vi "Configure IQ Attenuation.vi"(6 "Optimization Bandwidth (1 Msps)":dbl=1000000.0, 8 "error in (no error)":errorcluster, 9 "Manual Level (0.4 V)":dbl=0.4, 10 "I/Q Input Level Method (0: Default)":u16(ring) items=["Default", "Manual", "Measurement"], 11 "VISA resource name":refnum<visa-resource-name>) -> (0 "error out":errorcluster, 3 "VISA resource name out":refnum<visa-resource-name>)   [LabVIEW 2014, in "Agilent PSG MXG Series.lvlib"]
doc: "Configures attenuation mode, attenuation level, external I/Q input level and bandwidth.\n\n<B>Notes:</B>\n(1) This VI is valid only in E8267C, E8267D."
uses:
  Agilent PSG MXG Series.lvlib
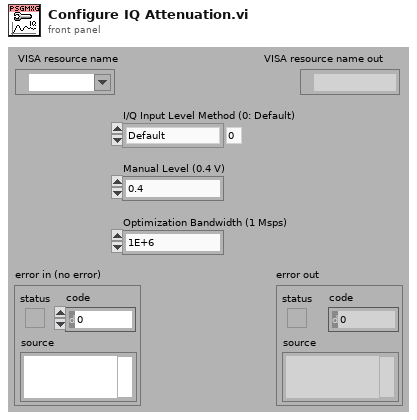
[diagram p1: front panel]
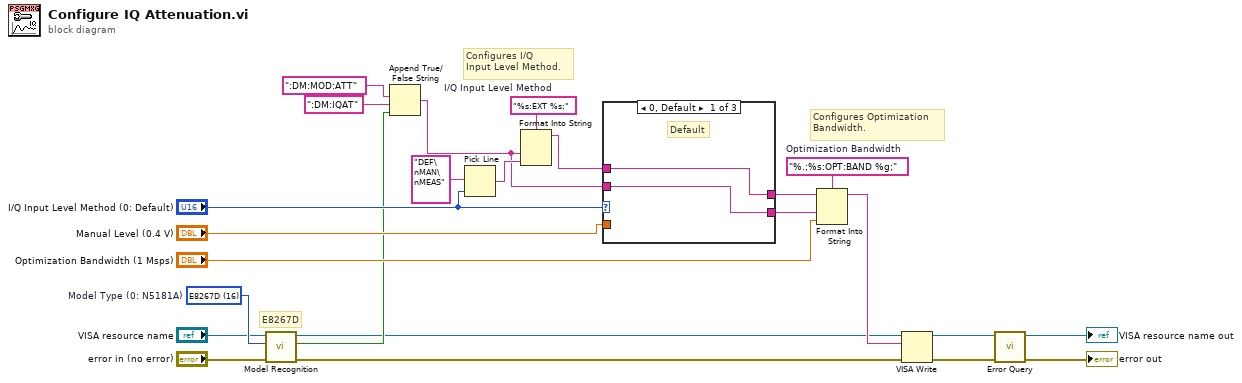
[diagram p0: block diagram]
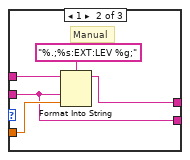
[diagram p2: hidden frame]
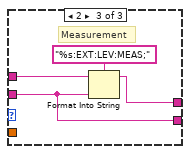
[diagram p3: hidden frame]
diagram:
  w8 = u16 16 items=["N5181A"=0, "N5182A"=1, "E8241A"=5, "E8244A"=6, "E8251A"=7, "E8254A"=8, "E8247C"=10, "E8257C"=11, "E8267C"=12, "E8257D"=15, "E8267D"=16]  # Model Type (0: N5181A)
  w20 = "%.;%s:OPT:BAND %g;"  # Optimization Bandwidth
  w24 = "%s:EXT %s;"  # I/Q Input Level Method
  # "Configures Optimization\nBandwidth."
  # "Configures I/Q\nInput Level Method."
  # "E8267D"
  n1 = call "Model Recognition.vi"("error in (no error)"="error in (no error)", "Model Type (0: N5181A)"=w8, "VISA resource name"="VISA resource name") -> ("error out"=w5:errorcluster, "Is Model Correct"=w7:bool, "VISA resource name out"=w6:refnum<visa-resource-name>)  [unwired: 6 out]
  n2 = Append True/False String(1:w7, 2:":DM:IQAT" ("false string"), 3:":DM:MOD:ATT" ("true string")) -> (0:w11:string)  [unwired: 1 out]
  n3 = Pick Line(multi-line string="DEF\nMAN\nMEAS", line index="I/Q Input Level Method (0: Default)") -> (output string=w14:string)  [unwired: 1 out]
  n4 = Format Into String(format string=w24, w11, w14) -> (resulting string=w22:string)  [unwired: 2 in, 1 out]
  n5 = case shown="0, Default" "I/Q Input Level Method (0: Default)" {
    tunnel: w22 -> [w26 w31 w34]
    tunnel: "Manual Level (0.4 V)" -> [_ w28 _]
    tunnel: [w26 w29 w33] -> w21
    tunnel: w11 -> [w25 w27 w32]
    tunnel: [w25 w27 w32] -> w10
    frame 0, Default {
      # "Default"
    }
    frame 1 {
      # "Manual"
      n6 = Format Into String(format string="%.;%s:EXT:LEV %g;", initial string=w31, w27, w28) -> (resulting string=w29:string)  [unwired: 1 in, 1 out]
    }
    frame 2 {
      # "Measurement"
      n7 = Format Into String(format string="%s:EXT:LEV:MEAS;", initial string=w34, w32) -> (resulting string=w33:string)  [unwired: 1 in, 1 out]
    }
  }
  n8 = Format Into String(format string=w20, initial string=w21, w10, "Optimization Bandwidth (1 Msps)") -> (resulting string=w19:string)  [unwired: 1 in, 1 out]
  n9 = VISA Write(VISA resource name=w6, write buffer=w19, error in (no error)=w5) -> (VISA resource name out=w18:refnum<visa-resource-name>, error out=w17:errorcluster)  [unwired: 1 out]
  n10 = call "Error Query.vi"("error in (no error)"=w17, "VISA resource name"=w18) -> ("error out"=→"error out":errorcluster, "VISA resource name out"=→"VISA resource name out":refnum<visa-resource-name>)  [unwired: 8 out]
